vi "Verify Core.vi"(8 "error in":errorcluster, 10 "Scrubbed String":string, 11 "Options in":refnum<class "Options.lvclass">) -> (0 "error out":errorcluster, 2 "Passed?":bool, 3 "String":string)   [LabVIEW 2020, in "Approval Tests.lvlib"]
uses:
  Approval Tests.lvlib
  Options/Options.lvclass
  Options/Options.lvclass/Options.ctl
  Options/Read Namer.vi
  Options/Read Naming Data.vi
  Options/Read Reporter.vi
  Options/Read Text Comparator.vi
  Namer/Namer.lvclass
  Naming Data/Naming Data.lvclass
  Reporter/Reporter.lvclass
  Text Comparator/Text Comparator.lvclass
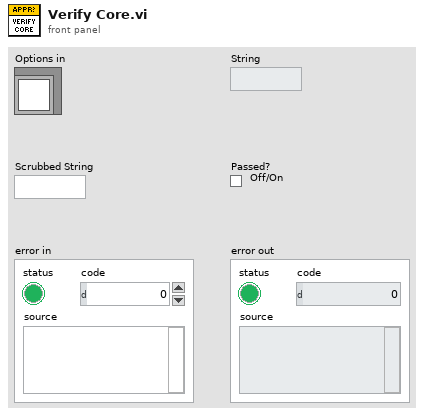
[diagram p1: front panel]
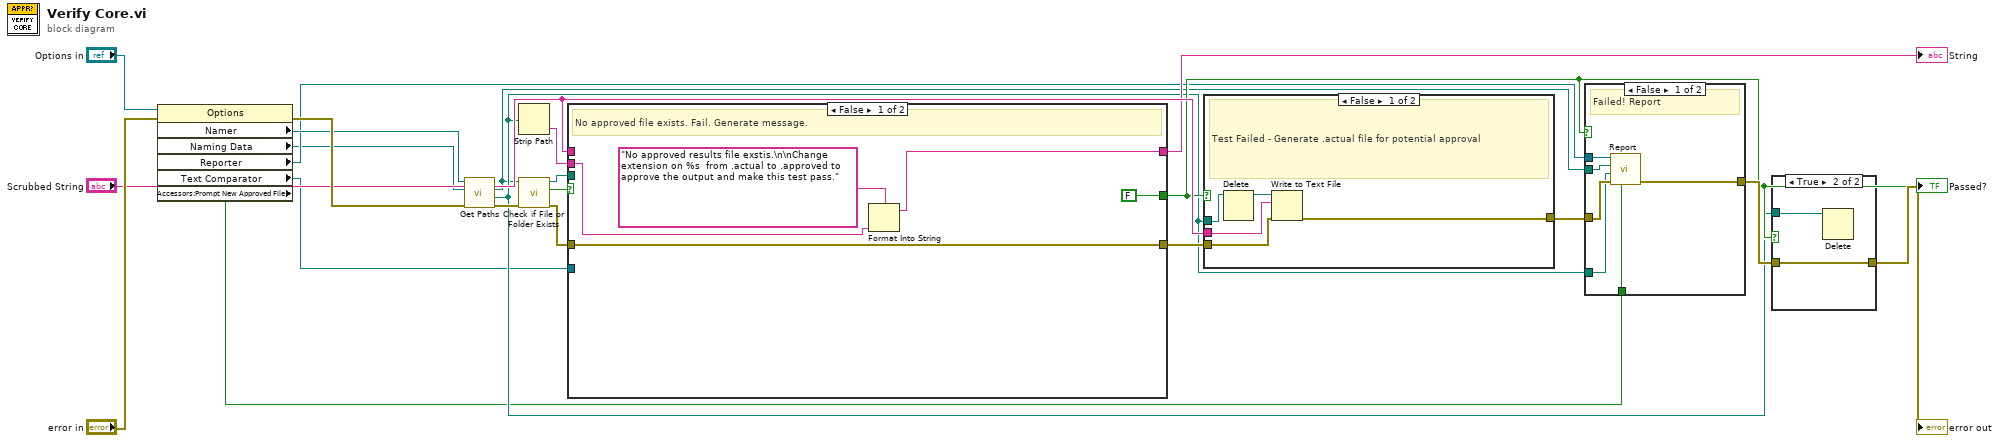
[diagram p0: block diagram]
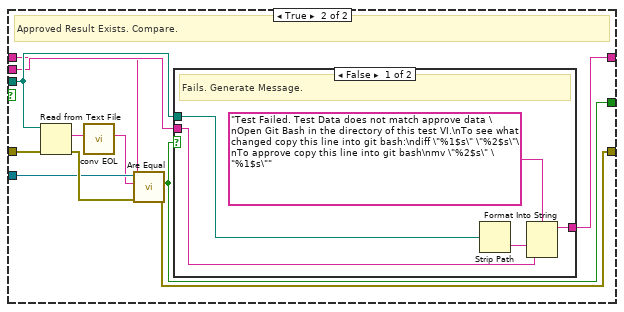
[diagram p5: hidden frame]
diagram:
  n1 = property class="Options"(reference="Options in", error in="error in") -> (error out=w15:errorcluster, "Namer"=w5:refnum<class "Namer.lvclass">, "Naming Data"=w1:refnum<class "Naming Data.lvclass">, "Reporter"=w2:refnum<class "Reporter.lvclass">, "Text Comparator"=w3:refnum<class "Text Comparator.lvclass">, "Accessors:Prompt New Approved File"=w4:bool)  [unwired: 1 out]
  n2 = call-dynamic "Get Paths.vi"("error in"=w15, "Naming Data"=w1, "Namer in"=w5) -> ("error out"=w22:errorcluster, "Received Path"=w8:path, "Approved Path"=w7:path)  [unwired: 5 in, 1 out]
  n3 = Strip Path(path=w8) -> (name=w13:string)  [unwired: 1 out]
  n4 = call <vilib>:"Check if File or Folder Exists.vi"("error in (no error)"=w22, "path"=w7) -> ("error out"=w19:errorcluster, "file or folder exists?"=w11:bool, "dup path"=w10:path)  [unwired: 7 in]
  n5 = case shown="False" w11 {
    tunnel: "Scrubbed String" -> [_ w29]
    tunnel: [w27 w36] -> w20
    tunnel: w19 -> [w27 w38]
    tunnel: w10 -> [_ w34]
    tunnel: [FALSE ("Passed?") w28] -> w9
    tunnel: [w23 w35] -> w12
    tunnel: w13 -> [w25 w33]
    tunnel: w3 -> [_ w31]
    frame False {
      # "No approved file exists. Fail. Generate message."
      n6 = Format Into String(format string="No approved results file exstis.\n\nChange extension on %s  from .actual to .approved to approve the output and make this test pass.", w25) -> (resulting string=w23:string)  [unwired: 2 in, 1 out]
    }
    frame True {
      # "Approved Result Exists. Compare."
      n7 = Read from Text File(file (use dialog)=w34, error in=w38) -> (text=w32:string, error out=w37:errorcluster)  [unwired: 2 in, 2 out]
      n8 = call "conv EOL.vi"("standard output in"=w32) -> ("result string"=w30:string)  [unwired: 10 in]
      n9 = call-dynamic "Are Equal.vi"("error in"=w37, "Received Text"=w29, "Approved Text"=w30, "Text Comparator in"=w31) -> ("error out"=w36:errorcluster, "Are Equal?"=w28:bool)  [unwired: 5 in, 1 out]
      n10 = case shown="False" w28 {
        tunnel: [w43 _] -> w35
        tunnel: w34 -> [w40 _]
        tunnel: w33 -> [w39 _]
        frame False {
          # "Fails. Generate Message."
          n11 = Strip Path(path=w40) -> (name=w41:string)  [unwired: 1 out]
          n12 = Format Into String(format string="Test Failed. Test Data does not match approve data \nOpen Git Bash in the directory of this test VI.\nTo see what changed copy this line into git bash:\ndiff \"%1$s\" \"%2$s\"\nTo approve copy this line into git bash\nmv \"%2$s\" \"%1$s\"", w41, w39) -> (resulting string=w43:string)  [unwired: 2 in, 1 out]
        }
        frame True {
          # "Passes. No Message Needed.."
        }
      }
    }
  }
  "Passed?" <- w9
  "String" <- w12
  n13 = case shown="False" w9 {
    tunnel: w20 -> [w47 w49]
    tunnel: [w48 w49] -> w21
    tunnel: w8 -> [w46 _]
    tunnel: "Scrubbed String" -> [w45 _]
    frame False {
      # "Test Failed - Generate .actual file for potential approval"
      n14 = Delete(path (use dialog)=w46) -> (deleted path=w44:path)  [unwired: 4 in, 2 out]
      n15 = Write to Text File(file (use dialog)=w44, text=w45, error in=w47) -> (error out=w48:errorcluster)  [unwired: 1 in, 2 out]
    }
    frame True {
      # "Passed - no need for .actual file"
    }
  }
  n16 = case shown="False" w9 {
    tunnel: w8 -> [w51 _]
    tunnel: w7 -> [w52 _]
    tunnel: w2 -> [w53 _]
    tunnel: w21 -> [w55 w56]
    tunnel: [w54 w56] -> w18
    tunnel: w4 -> [w50 _]
    frame False {
      # "Failed! Report"
      n17 = call "Report.vi"("Prompt to add new approved file to project? (T)"=w50, "error in"=w55, "Received"=w51, "Approved"=w52, "Reporter in"=w53) -> ("error out"=w54:errorcluster)  [unwired: 4 in, 2 out]
    }
    frame True {
      # "Passed - Nothing to Report"
    }
  }
  n18 = case shown="True" w9 {
    tunnel: w18 -> [w57 w59]
    tunnel: [w57 w59] -> w17
    tunnel: w8 -> [_ w58]
    frame False {
    }
    frame True {
      n19 = Delete(path (use dialog)=w58) -> ()  [unwired: 4 in, 3 out]
    }
  }
  "error out" <- w17
